vi "Actor Core.vi"(8 "error in":errorcluster, 11 "Detector Actor in":refnum<class "Detector Actor.lvclass">) -> (0 "error out":errorcluster, 3 "Actor out":refnum<class "Actor.lvclass">)   [LabVIEW 2019, in "Detector Actor.lvlib" / "Detector Actor.lvclass"]
doc: "(<B>Filename</B>: Actor Framework.lvlib:Actor.lvclass:Actor Core.vi)\n\nReceives messages to the actor, reacts to them, and initiates any error handling that may shut the actor down.\n\nDescendant classes may override this VI to append parallel tasks for the actor to complete while it handles messages. Overrides use the Call Parent Method node."
uses:
  Detector Actor.lvclass
  C:/Program Files (x86)/National Instruments/LabVIEW 2019/vi.lib/ActorFramework/Actor/Actor.lvclass
  <vilib>/ActorFramework/Actor/Actor.lvclass
  Detector Actor.lvclass/Detector Actor.ctl
  <vilib>/ActorFramework/Actor/Actor.lvclass/Actor.ctl
  Controller/Controller Messages/New Event Msg/New Event Msg.lvclass/New Event Msg.ctl
  <vilib>/ActorFramework/Message Enqueuer/Message Enqueuer.lvclass/Message Enqueuer.ctl
  <vilib>/ActorFramework/Message Enqueuer/Enqueue.vi
  Controller/Controller Messages/New Event Msg/New Event Msg.lvclass
  C:/Program Files (x86)/National Instruments/LabVIEW 2019/vi.lib/ActorFramework/Message/Message.lvclass
  <vilib>/ActorFramework/Message Priority Queue/Priority Enqueue.vi
  Sensors/Detector/Muon Detector.lvclass
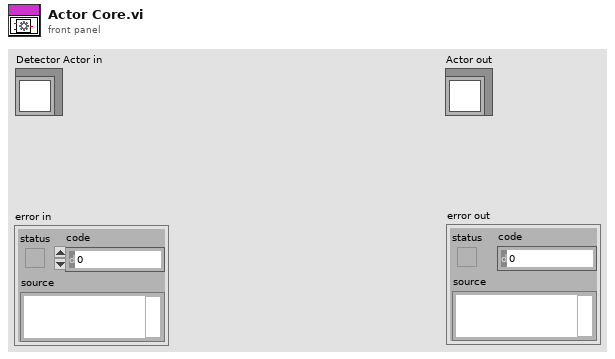
[diagram p1: front panel]
types:
  T1 = typedef "Muon Detector.lvclass/Event.ctl" = cluster{"Event Count":i32, "Device Timestamp (ms)":i32, "PC Timestamp":timestamp, "ADC Count":i32, "Event Type":u8}
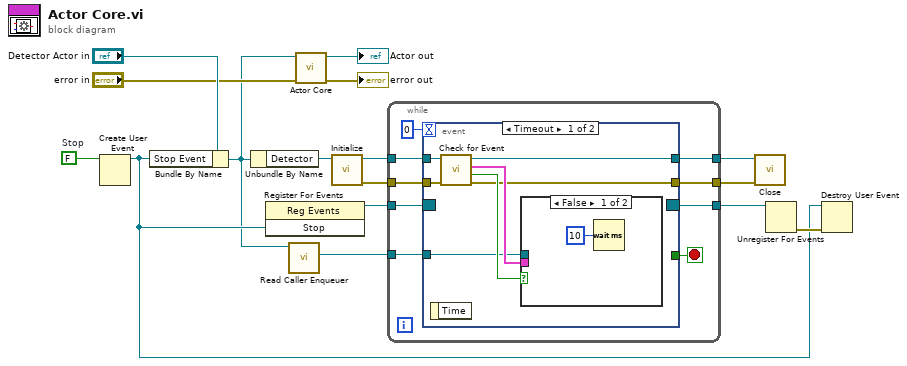
[diagram p0: block diagram]
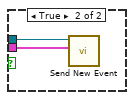
[diagram p2: hidden frame]
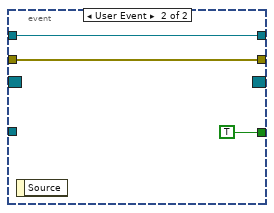
[diagram p3: hidden frame]
diagram:
  w7 = FALSE  # Stop
  n1 = Create User Event(user event datatype=w7) -> (user event=w3:refnum<user-event>)  [unwired: 1 in, 1 out]
  n2 = Bundle By Name(cluster="Detector Actor in", "Stop Event"=w3) -> (w2:refnum<class "Detector Actor.lvclass">)
  n3 = Unbundle By Name(w2) -> ("Detector"=w8:refnum<class "Muon Detector.lvclass">)
  n4 = register-events(w3) -> (reference out=w6:refnum<event-registration>)  [unwired: 2 in, 1 out]
  n5 = call <vilib>:"Read Caller Enqueuer.vi"("Actor"=w2) -> ("Caller Enqueuer"=w1:refnum<class "Message Enqueuer.lvclass">)  [unwired: 10 in]
  n6 = call-parent "Actor Core.vi"("error in"="error in", "Actor in"=w2) -> ("error out"=→"error out":errorcluster, "Actor out"=→"Actor out":refnum<class "Actor.lvclass">)  [unwired: 8 in]
  n7 = call-dynamic "Initialize.vi"("Muon Detector in"=w8) -> ("error out"=w11:errorcluster, "Muon Detector out"=w12:refnum<class "Muon Detector.lvclass">)  [unwired: 9 in]
  n8 = while {
    tunnel: w12 -> [w25]
    tunnel: w11 -> [w24]
    tunnel: [w23] -> w10
    tunnel: [w22] -> w9
    tunnel: w6 -> [w20]
    tunnel: [w19] -> w5
    tunnel: w1 -> [w17]
    stop <- w18 stop-if-true
    n9 = event shown="[0] Timeout" {
      selector: w20 -> [_ _]
      dyn-events: [_ _] -> w19
      timeout: 0 -> [_ _]
      tunnel: w25 -> [w30 w37]
      tunnel: w24 -> [w29 w36]
      tunnel: [w28 w37] -> w23
      tunnel: [w27 w36] -> w22
      tunnel: [_ TRUE] -> w18
      tunnel: w17 -> [w26 _]
      event Timeout {
        n10 = event-data() -> ()  [unwired: 1 in, 1 out]
        n11 = call "Check for Event.vi"("error in (no error)"=w29, "Muon Detector in"=w30) -> ("error out"=w27:errorcluster, "Valid?"=w32:bool, "Event"=w31:T1, "Muon Detector out"=w28:refnum<class "Muon Detector.lvclass">)  [unwired: 6 in]
        n12 = case shown="False" w32 {
          tunnel: w31 -> [_ w34]
          tunnel: w26 -> [_ w35]
          frame False {
            n13 = Wait (ms)(milliseconds to wait=u32 10) -> ()  [unwired: 1 out]
          }
          frame True {
            n14 = call "Send New Event.vi"("Event"=w34, "Message Enqueuer"=w35) -> ()  [unwired: 8 in, 2 out]
          }
        }
      }
      event User Event {
        n15 = event-data() -> ()  [unwired: 1 in, 1 out]
      }
    }
  }
  n16 = call-dynamic "Close.vi"("error in (no error)"=w9, "Muon Detector in"=w10) -> ()  [unwired: 8 in, 2 out]
  n17 = Unregister For Events(event registration refnum=w5) -> (error out=w4:errorcluster)  [unwired: 1 in]
  n18 = Destroy User Event(user event=w3, error in=w4) -> ()  [unwired: 1 out]
